vi "VCS Set Position Must.vi"(8 "error in (no error)":errorcluster, 10 "positionMust":i32, 11 "axis in":cluster{"keyHandle":u32, "nodeId":u16}={"keyHandle"=0, "nodeId"=1}) -> (0 "error out":errorcluster, 3 "axis out":cluster{"keyHandle":u32, "nodeId":u16}={"keyHandle"=0, "nodeId"=1})   [LabVIEW 2010]
doc: "<B>VCS Set Position Must</B> sets the new position demand value."
uses:
  Resources/EposCmd.dll
  Resources/EposCmd64.dll
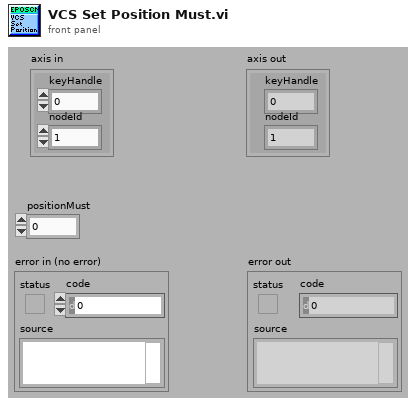
[diagram p1: front panel]
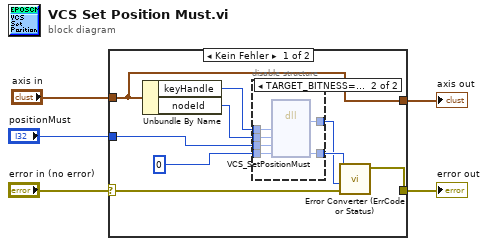
[diagram p0: block diagram]
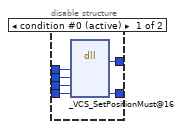
[diagram p2: hidden frame]
diagram:
  n1 = case shown="Kein Fehler" "error in (no error)" {
    selector: "error in (no error)" -> [w13 w28]
    tunnel: [w12 w28] -> w4
    tunnel: "positionMust" -> [w14 _]
    tunnel: "axis in" -> [w8 w27]
    tunnel: [w8 w27] -> w1
    frame No Error {
      n2 = Unbundle By Name(w8) -> ("keyHandle"=w10:u32, "nodeId"=w9:u16)
      n3 = disable-structure shown="TARGET_BITNESS==64" {
        disable-tunnel: w14 -> [w20 w26]
        disable-tunnel: [w19 w25] -> w11
        disable-tunnel: w10 -> [w18 w24]
        disable-tunnel: w9 -> [w17 w23]
        disable-tunnel: u32 0 ("pErrorCode") -> [w16 w22]
        disable-tunnel: [w15 w21] -> w6
        frame condition #0 (active) {
          n4 = dll-call lib="C:/Sources/LabView/maxon EPOS/Resources/EposCmd.*" fn="_VCS_SetPositionMust@16"("KeyHandle"=w18, "NodeId"=w17, "PositionMust"=w20, "pErrorCode"=w16) -> (w15:i32, "pErrorCode"=w19:u32)  [unwired: 6 in, 2 out]
        }
        frame condition #1 {
          n5 = dll-call lib="C:/setup/Resources/EposCmd64.*" fn="VCS_SetPositionMust" ("EposCmd.dll:_VCS_SetPositionMust@16")("KeyHandle"=w24, "NodeId"=w23, "PositionMust"=w26, "pErrorCode"=w22) -> ("Rückgabetyp"=w21:i32, "pErrorCode"=w25:u32)  [unwired: 6 in, 2 out]
        }
      }
      n6 = call "Error Converter (ErrCode or Status).vi"("error code"=w11, "return type"=w6, "error in (no error)"=w13) -> ("error out"=w12:errorcluster)  [unwired: 7 in]
    }
    frame Error {
    }
  }
  "error out" <- w4
  "axis out" <- w1
